vi "OCR_Create unique color list.vi"(8 "Error":errorcluster, 9 "Frame Color":u32(colorbox), 11 "Array":T1[](array[typedef])) -> (0 "Error Out":errorcluster, 3 "Duplicats Removed Out":T1[](array[typedef]))   [LabVIEW 2009]
uses:
  Controls/Cluster/Cluster_Text Color Set.ctl
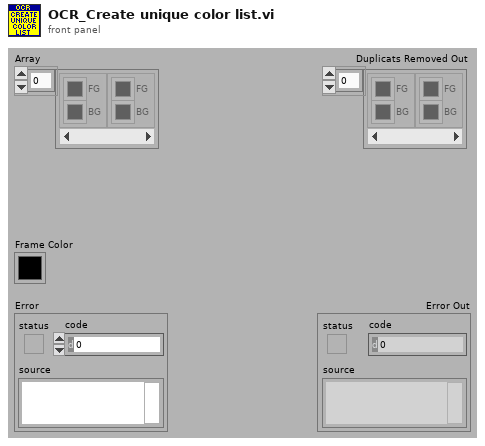
[diagram p1: front panel]
types:
  T1 = typedef "Cluster_Text Color Set.ctl" = cluster{"BG":u32, "FG":u32}
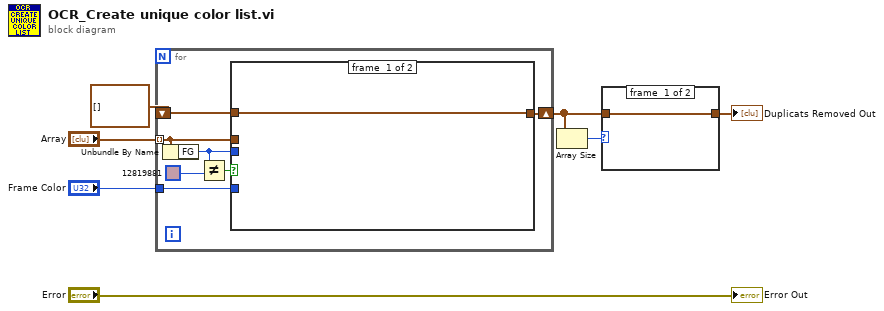
[diagram p0: block diagram]
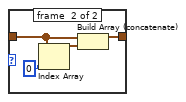
[diagram p2: hidden frame]
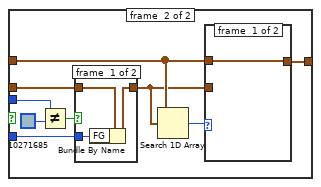
[diagram p3: hidden frame]
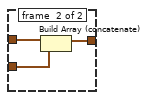
[diagram p4: hidden frame]
diagram:
  n1 = for {
    tunnel: "Array" -> [w12] mode=indexing
    shift-right: [w10] -> w3
    shift-left: T1[] [] -> [w11]
    tunnel: "Frame Color" -> [w8]
    n2 = Unbundle By Name(w12) -> ("FG"=w9:u32)
    n3 = Not Equal?(x=w9, y=u32 12819881) -> (x != y?=w13:bool)
    n4 = case shown="True" w13 {
      tunnel: w12 -> [_ w20]
      tunnel: w11 -> [w15 w18]
      tunnel: [w15 w24] -> w10
      tunnel: w9 -> [_ w23]
      tunnel: w8 -> [_ w19]
      frame #0 {
      }
      frame #1 {
        n5 = Not Equal?(x=w23, y=u32 10271685) -> (x != y?=w21:bool)
        n6 = case shown="False" w21 {
          tunnel: w20 -> [w31 w32]
          tunnel: [w30 w32] -> w17
          tunnel: w19 -> [w29 _]
          frame #0 {
            n7 = Bundle By Name(cluster=w31, "FG"=w29) -> (w30:T1)
          }
          frame #1 {
          }
        }
        n8 = Search 1D Array(1D array=w18, element=w17) -> (index of element=w16:i32)  [unwired: 1 in]
        n9 = case shown="..-1" w16 {
          tunnel: [w25 w28] -> w24
          tunnel: w18 -> [w25 w27]
          tunnel: w17 -> [_ w26]
          frame #0 {
          }
          frame #1 {
            n10 = Build Array (concatenate)(w27, w26) -> (w28:T1[])
          }
        }
      }
    }
  }
  n11 = Array Size(array=w3) -> (size(s)=w1:i32)
  n12 = case shown="..1" w1 {
    tunnel: w3 -> [w33 w36]
    tunnel: [w33 w34] -> w2
    frame #0 {
    }
    frame #1 {
      n13 = Index Array(array=w36, index=0) -> (element=w35:T1)
      n14 = Build Array (concatenate)(w36, w35) -> (w34:T1[])
    }
  }
  "Duplicats Removed Out" <- w2
  "Error Out" <- "Error"
